vi "Model - Init.vi"(8 "error in (no error)":errorcluster) -> (0 "error out":errorcluster, 3 "View Model":T1)   [LabVIEW 2017]
doc: "Initialize central data/events storage of MVC."
uses:
  Controls/View Model.ctl
  Controls/Shared Model.ctl
  Error Handler/Controls/Error Model.ctl
  Error Handler/Controls/Error Message.ctl
  Error Handler/Controls/Error Level.ctl
  Configuration/Controls/Database Model.ctl
  Configuration/Controls/Database Message.ctl
  Configuration/Controls/Database Command.ctl
  Configuration/Controls/Database Overhead.ctl
  Configuration/Controls/Database Status.ctl
  Configuration/Controls/Database Record.ctl
  Configuration/Controls/Database - Rule Record.ctl
  Controller/Controls/CNTRLR - Wash Step.ctl
  Controller/Controls/CNTRLR - Position.ctl
  Controller/Controls/CNTRLR - Model.ctl
  Controller/Controls/CNTRLR - Message.ctl
  Controller/Controls/CNTRLR - Command.ctl
  Controller/Controls/CNTRLR - Overhead.ctl
  Controller/Controls/CNTRLR - State.ctl
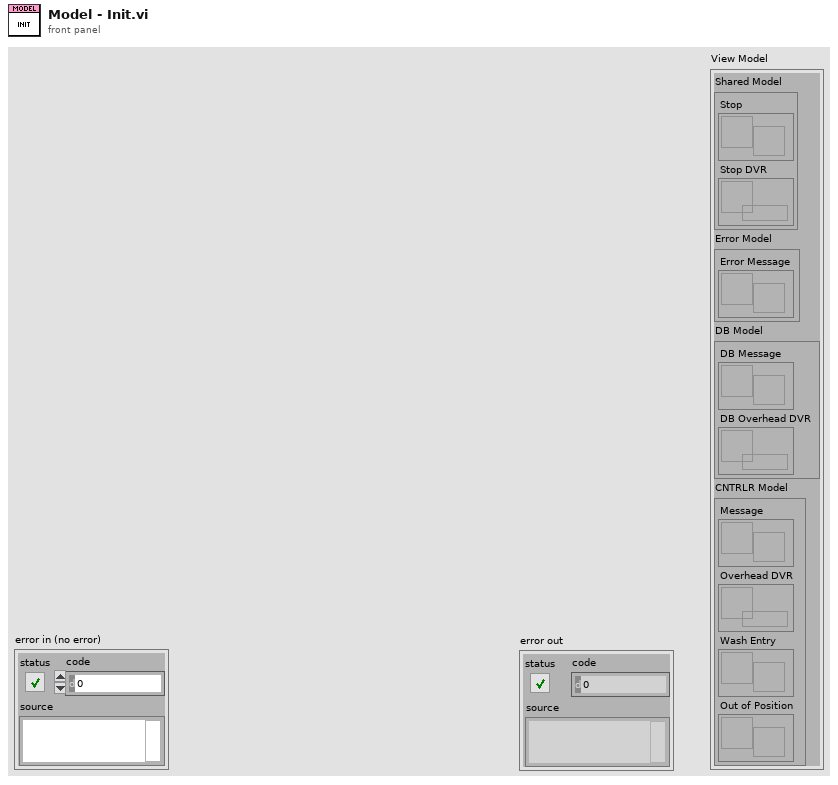
[diagram p1: front panel]
types:
  T1 = typedef "View Model.ctl" = cluster{"Shared Model":T2, "Error Model":T3, "DB Model":T4, "CNTRLR Model":T5}
  T2 = typedef "Shared Model.ctl" = cluster{"Stop":refnum<user-event>, "Stop DVR":refnum<data-value>}
  T3 = typedef "Error Model.ctl" = cluster{"Error Message":refnum<user-event>}
  T4 = typedef "Database Model.ctl" = cluster{"DB Message":refnum<user-event>, "DB Overhead DVR":refnum<data-value>}
  T5 = typedef "CNTRLR - Model.ctl" = cluster{"Message":refnum<user-event>, "Overhead DVR":refnum<data-value>, "Wash Entry":refnum<user-event>, "Out of Position":refnum<user-event>}
  T6 = typedef "CNTRLR - Overhead.ctl" = cluster{"Vehicle Position":T7, "Current State":T8, "Next State":T8, "Wash Cycle":T9[], "Current Wash Step":T10, "Time Remaining":dbl, "Last Step?":bool}
  T7 = typedef "CNTRLR - Position.ctl" = enum16{"Entry", "Station 1", "Station 2", "Station 3", "Exit"}
  T8 = typedef "CNTRLR - State.ctl" = enum16{"Initial", "Wait for Start", "Start State", "Wait for Vehicle Position", "Wash Step Execution", "Wash Step/Cycle Complete", "Wash Exit", "Wash Abort/Terminate"}
  T9 = typedef "Database Record.ctl" = cluster{"Wash Step":string, "Station":string, "Step Duration":u32}
  T10 = typedef "CNTRLR - Wash Step.ctl" = enum16{"Under Body Wash", "Bug Remover", "Pre-Soak", "High Pressure Wash", "Low Pressure Wax", "Spot Free Rinse", "Tire Shine Foam", "Air Dry", "None"}
  T11 = typedef "CNTRLR - Message.ctl" = cluster{"CMD":T12, "Data":variant}
  T12 = typedef "CNTRLR - Command.ctl" = enum16{"Idle", "Start Car Wash", "Error", "Stop"}
  T13 = typedef "Database Overhead.ctl" = cluster{"DB Status":T14, "DB Records":T9[], "Steps Rules":T15[], "Current Step Record":T15}
  T14 = typedef "Database Status.ctl" = enum16{"Unlocked", "Locked"}
  T15 = typedef "Database - Rule Record.ctl" = cluster{"Wash Step":T10, "Station":T7, "Step Timing":dbl}
  T16 = typedef "Database Message.ctl" = cluster{"DB Command":T17, "DB Data":variant}
  T17 = typedef "Database Command.ctl" = enum16{"Read Records", "Query Timing", "Insert New Data", "Update Data"}
  T18 = typedef "Error Message.ctl" = cluster{"Error Level":T19, "Error Data":variant}
  T19 = typedef "Error Level.ctl" = enum16{"Minor Error", "Wash Cycle Error", "System Error"}
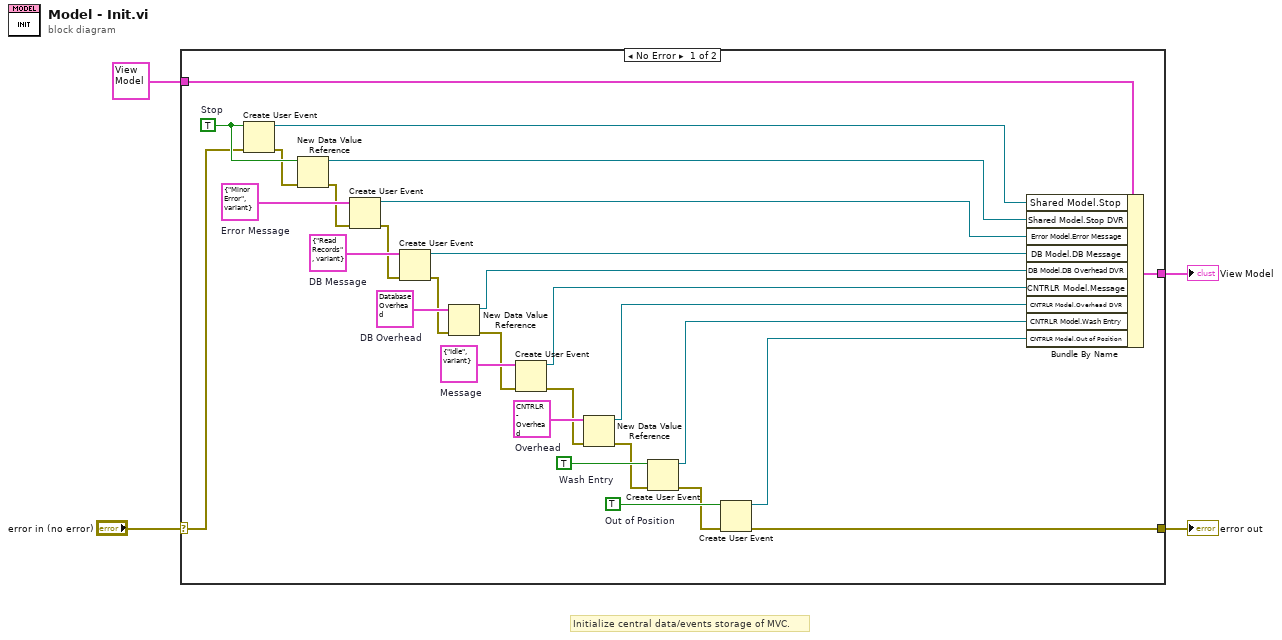
[diagram p0: block diagram]
diagram:
  # "Initialize central data/events storage of MVC."
  n1 = case shown="No Error" "error in (no error)" {
    selector: "error in (no error)" -> [w29 w35]
    tunnel: [w14 w35] -> w3
    tunnel: T1 {"Shared Model"={"Stop"=refnum, "Stop DVR"=refnum}, "Error Model"={"Error Message"=refnum}, "DB Model"={"DB Message"=refnum, "DB Overhead DVR"=refnum}, "CNTRLR Model"={"Message"=refnum, "Overhead DVR"=refnum, "Wash Entry"=refnum, "Out of Position"=refnum}} ("View Model") -> [w33 w34]
    tunnel: [w32 w34] -> w1
    frame No Error {
      w17 = TRUE  # Out of Position
      w18 = TRUE  # Wash Entry
      w21 = T6 {"Vehicle Position"=enum."Entry", "Current State"=enum."Initial", "Next State"=enum."Initial", "Wash Cycle"=[], "Current Wash Step"=enum."Under Body Wash", "Time Remaining"=0.0, "Last Step?"=FALSE}  # Overhead
      w22 = T11 {"CMD"=enum."Idle", "Data"=variant}  # Message
      w25 = T13 {"DB Status"=enum."Unlocked", "DB Records"=[], "Steps Rules"=[], "Current Step Record"={"Wash Step"=enum."Under Body Wash", "Station"=enum."Entry", "Step Timing"=0.0}}  # DB Overhead
      w26 = T16 {"DB Command"=enum."Read Records", "DB Data"=variant}  # DB Message
      w28 = T18 {"Error Level"=enum."Minor Error", "Error Data"=variant}  # Error Message
      w31 = TRUE  # Stop
      n2 = Create User Event(user event datatype=w31, error in=w29) -> (user event=w13:refnum<user-event>, error out=w30:errorcluster)
      n3 = New Data Value Reference(data value=w31, error in=w30) -> (data value reference=w12:refnum<data-value>, error out=w27:errorcluster)
      n4 = Create User Event(user event datatype=w28, error in=w27) -> (user event=w11:refnum<user-event>, error out=w24:errorcluster)
      n5 = Create User Event(user event datatype=w26, error in=w24) -> (user event=w10:refnum<user-event>, error out=w23:errorcluster)
      n6 = New Data Value Reference(data value=w25, error in=w23) -> (data value reference=w9:refnum<data-value>, error out=w20:errorcluster)
      n7 = Create User Event(user event datatype=w22, error in=w20) -> (user event=w8:refnum<user-event>, error out=w19:errorcluster)
      n8 = New Data Value Reference(data value=w21, error in=w19) -> (data value reference=w7:refnum<data-value>, error out=w16:errorcluster)
      n9 = Create User Event(user event datatype=w18, error in=w16) -> (user event=w6:refnum<user-event>, error out=w15:errorcluster)
      n10 = Create User Event(user event datatype=w17, error in=w15) -> (user event=w5:refnum<user-event>, error out=w14:errorcluster)
      n11 = Bundle By Name(cluster=w33, "Shared Model.Stop"=w13, "Shared Model.Stop DVR"=w12, "Error Model.Error Message"=w11, "DB Model.DB Message"=w10, "DB Model.DB Overhead DVR"=w9, "CNTRLR Model.Message"=w8, "CNTRLR Model.Overhead DVR"=w7, "CNTRLR Model.Wash Entry"=w6, "CNTRLR Model.Out of Position"=w5) -> (w32:T1)
    }
    frame Error {
    }
  }
  "error out" <- w3
  "View Model" <- w1
